vi "Set Diverter.vi"(8 "error in (no error)":errorcluster, 9 "Diverter Port":T1, 10 "Diverter Location":T2, 11 "Simulated in":refnum<class "Simulated.lvclass">) -> (0 "error out":errorcluster, 1 "Diverter Port out":T1, 3 "Simulated out":refnum<class "Simulated.lvclass">)   [LabVIEW 2019, in "Simulated.lvclass"]
uses:
  Simulated.lvclass
  SpectraPro-LabVIEW-Driver/Libraries/Types/Diverter Location.ctl
  SpectraPro-LabVIEW-Driver/Libraries/Types/Diverter Port.ctl
  SpectraPro-LabVIEW-Driver/SpectraPro.lvlib
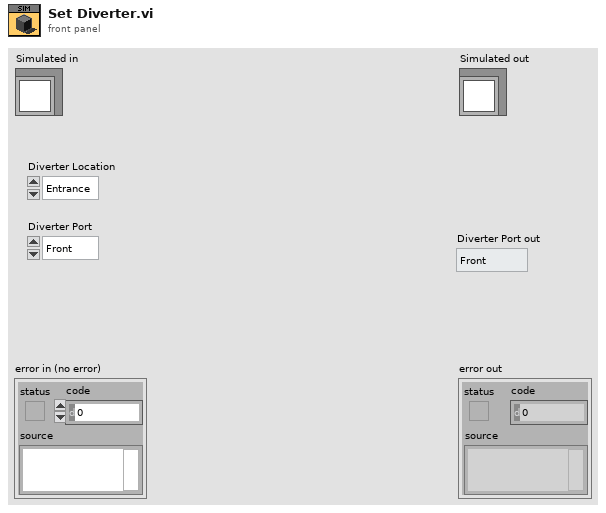
[diagram p1: front panel]
types:
  T1 = typedef "SpectraPro.lvlib/Diverter Port.ctl" = enum16{"Front", "Side"}
  T2 = typedef "Diverter Location.ctl" = enum16{"Entrance", "Exit"}
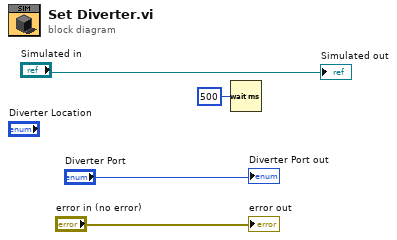
[diagram p0: block diagram]
diagram:
  n1 = Wait (ms)(milliseconds to wait=u32 500) -> ()  [unwired: 1 out]
  "error out" <- "error in (no error)"
  "Simulated out" <- "Simulated in"
  "Diverter Port out" <- "Diverter Port"
